vi "Start.vi"(0 "eye scan in":refnum<class "niHighSpeedSerial N Point Eye Scan v1 Host.lvclass">, 11 "error in":errorcluster) -> (4 "eye scan out":refnum<class "niHighSpeedSerial N Point Eye Scan v1 Host.lvclass">, 15 "error out":errorcluster)   [LabVIEW 2014, in "niHighSpeedSerial N Point Eye Scan v1 Host.lvclass"]
doc: "Moves the session into the Running state and begins measuring the first point.\n\n<B>Input Parameters</B>\n\n<B>eye scan in</B> Takes in a reference to your session from the previous VI.\n\n<B>error in</B> describes error conditions that occur before this node runs. This input provides standard 'error in' functionality.\n\n<B>Output Parameters</B>\n\n<B>eye scan out</B> passes a reference to your session to the next VI.\n\n<B>error out</B> contains error information. This output provides standard 'error out' functionality."
uses:
  <instrlib>/niHighSpeedSerial/Eye Scan/v1/Host/Impl/N Point Eye Scan/niHighSpeedSerial N Point Eye Scan v1 Host.lvclass
  <instrlib>/niHighSpeedSerial/Eye Scan/v1/Host/Impl/N Point Eye Scan/niHighSpeedSerial N Point Eye Scan v1 Host.lvclass/niHighSpeedSerial N Point Eye Scan v1 Host.ctl
  <instrlib>/niHighSpeedSerial/Eye Scan/v1/Host/Eye Scan/niHighSpeedSerial Eye Scan v1 Host.lvclass
  <instrlib>/niHighSpeedSerial/Eye Scan/v1/Host/Impl/N Pt Iter/niHighSpeedSerial N Point Eye Scan Point Iterator v1 Host.lvclass
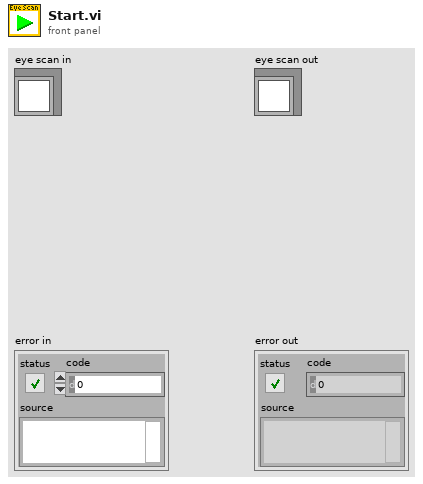
[diagram p1: front panel]
types:
  T1 = typedef "N Point Eye Scan v1 Host.lvclass/Private Data.ctl" = cluster{"array of points to measure":T2[], "n point eye scan point iterator":refnum<class "niHighSpeedSerial N Point Eye Scan Point Iterator v1 Host.lvclass">}
  T2 = typedef "niHighSpeedSerial Eye Scan Common v1 Host.lvlib/Point Offsets.ctl" = cluster{"horizontal offset":i16, "vertical offset":i8}
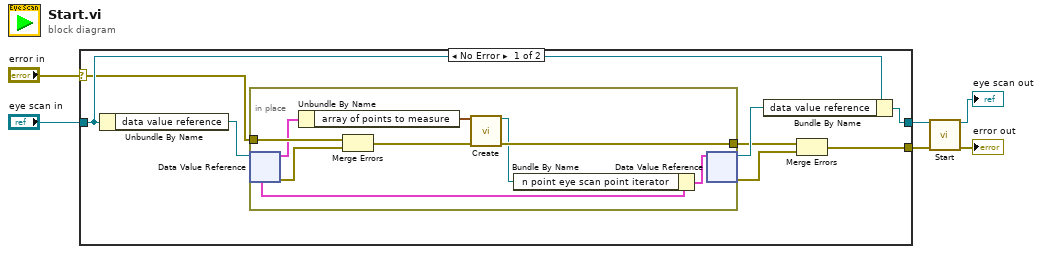
[diagram p0: block diagram]
diagram:
  n1 = case shown="No Error" "error in" {
    selector: "error in" -> [w7 w24]
    tunnel: [w10 w24] -> w1
    tunnel: [w12 w23] -> w4
    tunnel: "eye scan in" -> [w8 w23]
    frame No Error {
      n2 = Unbundle By Name(w8) -> ("data value reference"=w14:refnum<data-value>)
      n3 = in-place {
        in-place-border: w7 -> [w21]
        in-place-border: [w18] -> w9
        n4 = in-place-dvr #1(w14) -> (w17:T1, w20:errorcluster)
        n5 = Unbundle By Name(w17) -> ("array of points to measure"=w22:T2[])
        n6 = Merge Errors(w21, w20) -> (w19:errorcluster)
        n7 = call <instrlib>:"Create.vi"("array of point offsets"=w22, "error in"=w19) -> ("eye scan point iterator out"=w16:refnum<class "niHighSpeedSerial N Point Eye Scan Point Iterator v1 Host.lvclass">, "error out"=w18:errorcluster)  [unwired: 12 in]
        n8 = Bundle By Name(cluster=w17, "n point eye scan point iterator"=w16) -> (w15:T1)
        n9 = in-place-dvr #1(w15) -> (w13:refnum<data-value>, w11:errorcluster)
      }
      n10 = Bundle By Name(cluster=w8, "data value reference"=w13) -> (w12:refnum<class "niHighSpeedSerial N Point Eye Scan v1 Host.lvclass">)
      n11 = Merge Errors(w9, w11) -> (w10:errorcluster)
    }
    frame Error {
    }
  }
  n12 = call-parent "Start.vi"("eye scan in"=w4, "error in"=w1) -> ("eye scan out"=→"eye scan out":refnum<class "niHighSpeedSerial N Point Eye Scan v1 Host.lvclass">, "error out"=→"error out":errorcluster)  [unwired: 12 in]
